vi "GUI_digitizerONLY.vi"() -> ()   [LabVIEW 2013]
uses:
  shared programs/GUI_Template/GUI_master/tcp_new_data_event.ctl
  shared programs/GUI_Template/GUI_master/tcp new data cluster.ctl
panel:
  in  "Digitizer Traces":T1
  out "error IO 2":errorcluster
  in  "insert tag":bool=TRUE
  out "tcp data event":T2
  in  "GUIdevice 7":string="TS-digitizer-1"
  in  "stop":bool
  # "TEST STAND GRAPHICAL USER INTERFACE"
  # "- SCREEN 1"
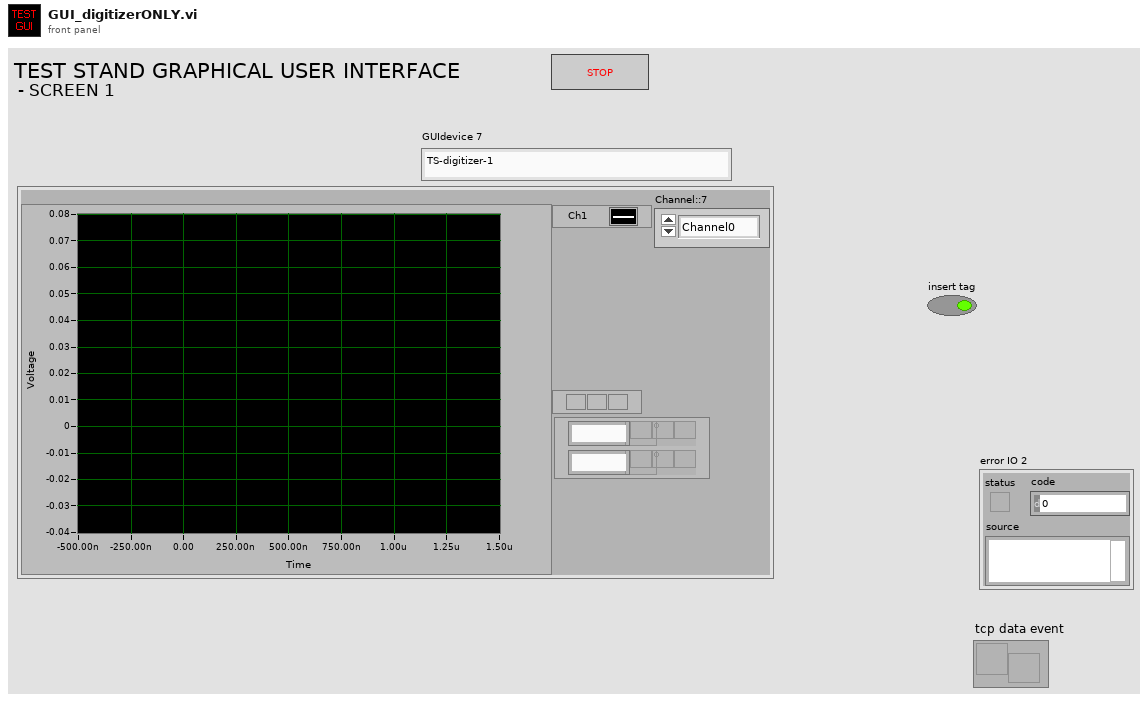
[diagram p1: front panel]
types:
  T1 = cluster{"Channel::7":enum16{"Channel0", "Channel1"}, "scopeTraceGUI::7":waveform(dbl)[]}
  T2 = typedef "tcp_new_data_event.ctl" = refnum<user-event>
  T3 = typedef "tcp new data cluster.ctl" = cluster{"EventEnum":enum16{"new data", "connection status update"}, "Device name":string}
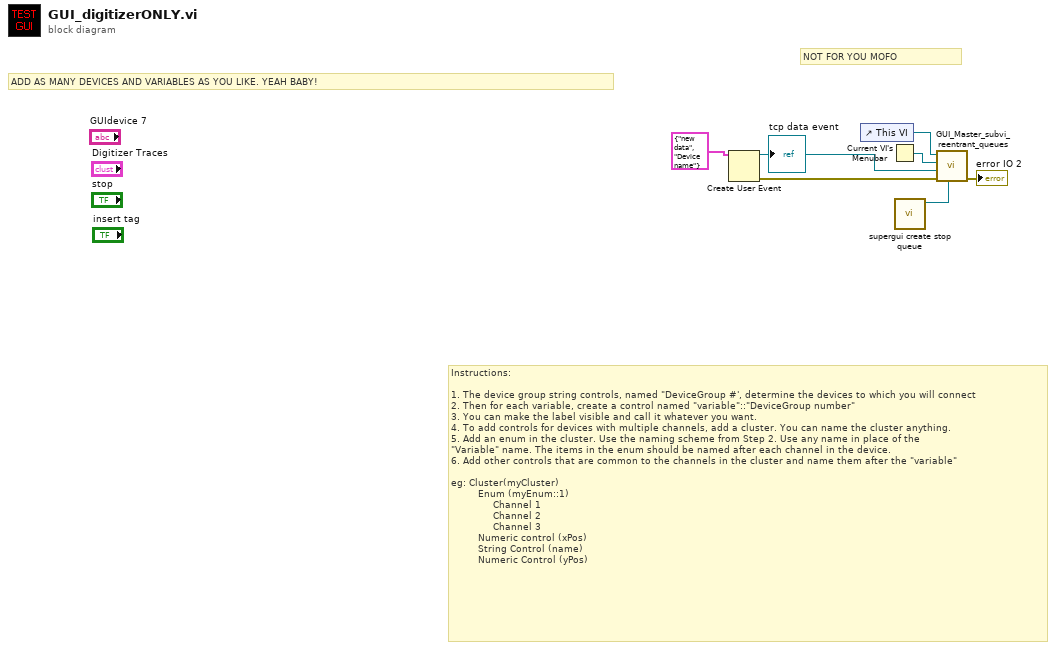
[diagram p0: block diagram]
diagram:
  # "Instructions:\n\n1. The device group string controls, named \"DeviceGroup #', determine the devices to which you will connect\n2. Then for each variable, create a control named \"variable\"::\"DeviceGroup number\"\n3. You can make the label visible and call it whatever you want.\n4. To add controls for devices with multiple channels, add a cluster. You can name the cluster anything.\n5. Add an enum in the cluster. Use the naming scheme from Step 2. Use any name in place of the \n\"Variable\" name. The items in the enum should be named after each channel in the device. \n6. Add other controls that are common to the channels in the cluster and name them after the \"variable\"\n\neg: Cluster(myCluster)\n         Enum (myEnum::1)\n              Channel 1 \n              Channel 2\n              Channel 3\n         Numeric control (xPos)\n         String Control (name)\n         Numeric Control (yPos)"
  # "ADD AS MANY DEVICES AND VARIABLES AS YOU LIKE. YEAH BABY!"
  # "NOT FOR YOU MOFO"
  n1 = Create User Event(user event datatype=T3 {"EventEnum"=enum."new data", "Device name"="Device name"} ("New Event")) -> (user event=w7:refnum<user-event>, error out=w6:errorcluster)  [unwired: 1 in]
  "tcp data event" <- w7
  n2 = control-ref of="This VI"() -> (w3:refnum<vi>)
  n3 = Current VI's Menubar() -> (w4:refnum<k9>)
  n4 = call "supergui create stop queue.vi"() -> ("STOP Queue out"=w1:refnum<queue>)  [unwired: 11 in]
  n5 = call "GUI_Master_subvi_reentrant_queues.vi"("STOP Queue in"=w1, "error in (no error)"=w6, "tcp data event"=w7, "Caller menu reference"=w4, "Caller VI ref"=w3) -> ("error out"=→"error IO 2":errorcluster)  [unwired: 6 in]
